vi "Aperture2String.vi"(7 "aperture":enum32{"Item 0", "Item 1", "Item 2", "Item 3"}(ring)) -> (8 "String":string)   [LabVIEW 2022 SP3]
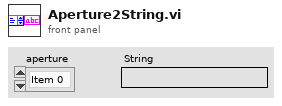
[diagram p1: front panel]
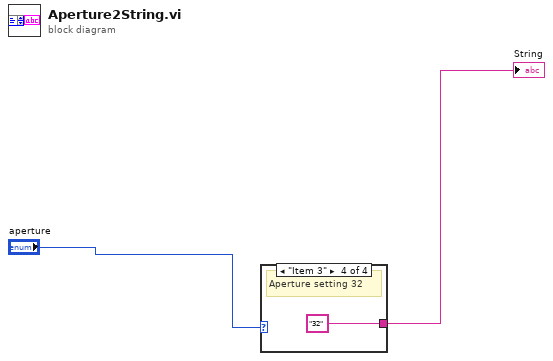
[diagram p0: block diagram]
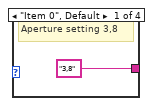
[diagram p2: hidden frame]
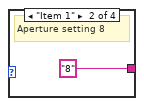
[diagram p3: hidden frame]
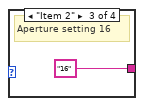
[diagram p4: hidden frame]
diagram:
  n1 = case shown="\"Item 3\"" "aperture" {
    tunnel: ["3,8" "8" "16" "32"] -> w2
    frame "Item 0", Default {
      # "Aperture setting 3,8"
    }
    frame "Item 1" {
      # "Aperture setting 8"
    }
    frame "Item 2" {
      # "Aperture setting 16"
    }
    frame "Item 3" {
      # "Aperture setting 32"
    }
  }
  "String" <- w2
